vi "String Array to Entries.vi"(11 "String Array in":string[][](array[string])) -> (0 "Total Duration":dbl, 1 "3-Entries":T1[](array[typedef]), 2 "2-Entries":T1[](array[typedef]), 3 "1-Entries":T1[](array[typedef]))   [LabVIEW 2019, in "Muon Data Post-Processing.lvlib"]
uses:
  Muon Data Post-Processing.lvlib
  File Entry.ctl
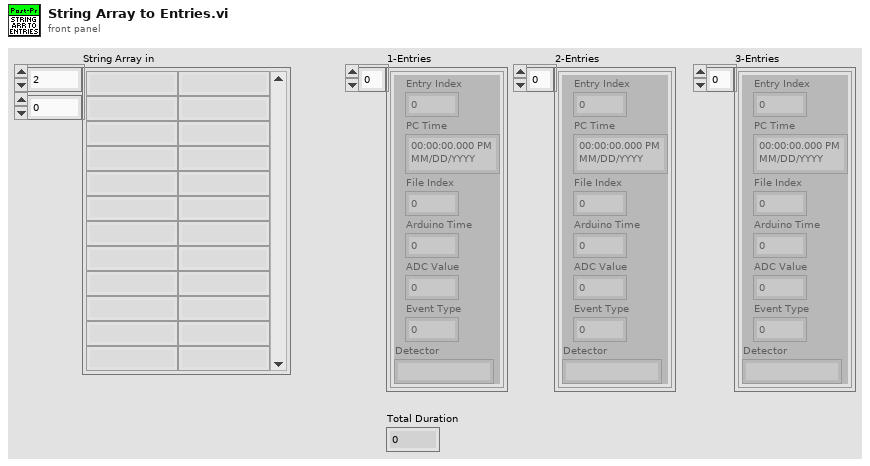
[diagram p1: front panel]
types:
  T1 = typedef "Muon Data Post-Processing.lvlib/File Entry.ctl" = cluster{"Entry Index":i32, "PC Time":timestamp, "File Index":i32, "Arduino Time":i32, "ADC Value":i32, "Event Type":i32, "Detector":string}
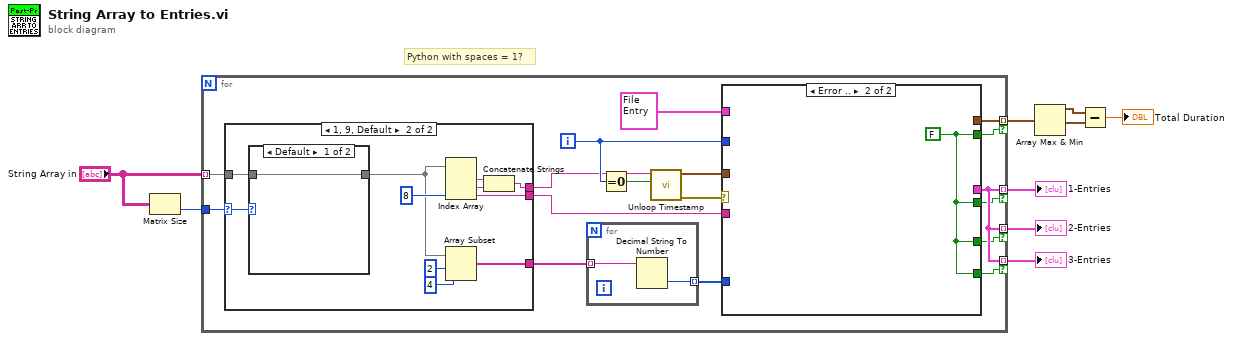
[diagram p0: block diagram]
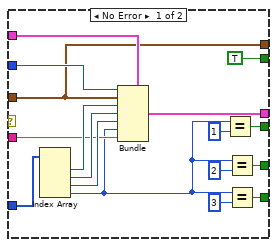
[diagram p2: hidden frame]
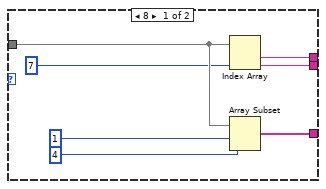
[diagram p3: hidden frame]
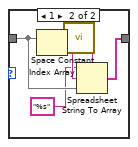
[diagram p4: hidden frame]
diagram:
  # "Python with spaces = 1?"
  n1 = Matrix Size(0:"String Array in") -> (2:w1:i32)  [unwired: 1 out]
  n2 = for {
    tunnel: "String Array in" -> [w26] mode=indexing
    tunnel: [w22] -> w9 mode=indexing if=w21
    tunnel: [w22] -> w8 mode=indexing if=w20
    tunnel: [w22] -> w7 mode=indexing if=w19
    tunnel: [w11] -> w6 mode=indexing if=w10
    tunnel: w1 -> [w14]
    i -> [w18]
    n3 = case shown="1, 9, Default" w14 {
      selector: w14 -> [_ w54]
      tunnel: w26 -> [w51 w52]
      tunnel: [w48 w60] -> w25
      tunnel: [w47 w59] -> w23
      tunnel: [w45 w55] -> w16
      frame 8 {
        n4 = Index Array(array=w51, index #2=7 ("index")) -> (element #1=w45:string, element #2=w47:string)  [unwired: 1 in]
        n5 = Array Subset(array=w51, index=1, length=4) -> (w48:string[])
      }
      frame 1, 9, Default {
        n6 = case shown="Default" w54 {
          tunnel: [w63 w67] -> w53
          tunnel: w52 -> [w63 w65]
          frame Default {
          }
          frame 1 {
            n7 = Index Array(array=w65) -> (element=w68:string)  [unwired: 1 in]
            n8 = call <vilib>:"Space Constant.vi"() -> ("String"=w66:string)
            n9 = Spreadsheet String To Array(delimiter (Tab)=w66, format string="%s", spreadsheet string=w68, array type (2D Dbl)=w65) -> (array=w67:string[])
          }
        }
        n10 = Index Array(array=w53, index #3=8 ("index")) -> (element #1=w57:string, element #2=w56:string, element #3=w59:string)  [unwired: 2 in]
        n11 = Array Subset(array=w53, index=2, length=4) -> (w60:string[])
        n12 = Concatenate Strings(w57, w56) -> (w55:string)
      }
    }
    n13 = for {
      tunnel: w25 -> [w69] mode=indexing
      tunnel: [w70] -> w24 mode=indexing
      n14 = Decimal String To Number(string=w69) -> (number=w70:i32)  [unwired: 2 in, 1 out]
    }
    n15 = Equal To 0?(x=w18) -> (x = 0?=w17:bool)
    n16 = call "Unloop Timestamp.vi"("Initialize?"=w17, "Time String"=w16) -> ("error IO"=w13:errorcluster, "Corrected Time Stamp"=w15:timestamp)  [unwired: 8 in]
    n17 = case shown="Error .." w13 {
      tunnel: w24 -> [w43 _]
      tunnel: w23 -> [w39 _]
      tunnel: T1 {"Entry Index"=0, "PC Time"=timestamp(0 s since 1904-01-01), "File Index"=0, "Arduino Time"=0, "ADC Value"=0, "Event Type"=0, "Detector"=""} ("cluster") -> [w38 _]
      tunnel: [w36 _] -> w22
      tunnel: [w35 w44] -> w21
      tunnel: [w32 w44] -> w20
      tunnel: [w31 w44] -> w19
      tunnel: w18 -> [w29 _]
      tunnel: w15 -> [w28 _]
      tunnel: [w28 _] -> w11
      tunnel: [TRUE w44] -> w10
      frame No Error {
        n18 = Index Array(array=w43) -> (element #1=w42:i32, element #2=w41:i32, element #3=w40:i32, element #4=w30:i32)  [unwired: 4 in]
        n19 = Bundle(cluster=w38, "Entry Index"=w29, "PC Time"=w28, "File Index"=w42, "Arduino Time"=w41, "ADC Value"=w40, "Event Type"=w30, "Detector"=w39) -> (w36:T1)
        n20 = Equal?(x=w30, y=1 ("x")) -> (x = y?=w35:bool)
        n21 = Equal?(x=w30, y=2 ("x")) -> (x = y?=w32:bool)
        n22 = Equal?(x=w30, y=3 ("x")) -> (x = y?=w31:bool)
      }
      frame Error {
        w44 = FALSE
      }
    }
  }
  "1-Entries" <- w9
  "2-Entries" <- w8
  "3-Entries" <- w7
  n23 = Array Max & Min(array=w6) -> (max value=w5:timestamp, min value=w4:timestamp)  [unwired: 2 out]
  n24 = Subtract(x=w5, y=w4) -> (x-y=→"Total Duration":dbl)
